vi "Static Read.vi"(8 "error in (no error)":errorcluster, 11 "Abs_Single Float in":refnum<class "Abs_Single Float.lvclass">) -> (0 "error out":errorcluster, 2 "Value":sgl, 3 "Abs_Single Float out":refnum<class "Abs_Single Float.lvclass">)   [LabVIEW 2021, in "Abs_Single Float.lvclass"]
uses:
  Abs_Single Float.lvclass
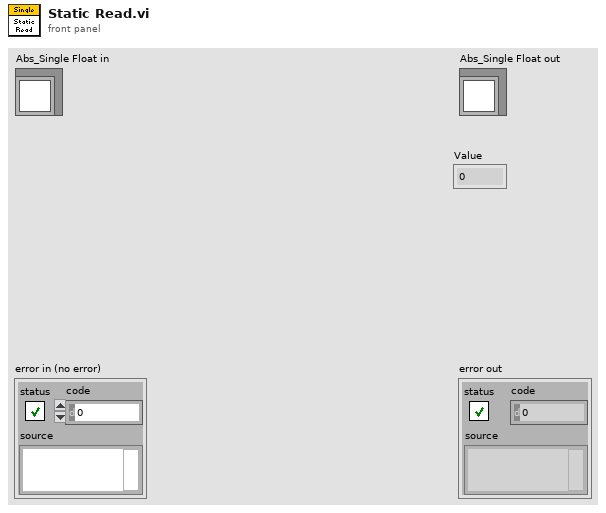
[diagram p1: front panel]
types:
  T1 = typedef "Abs_Single Float.lvclass/Type.ctl" = sgl
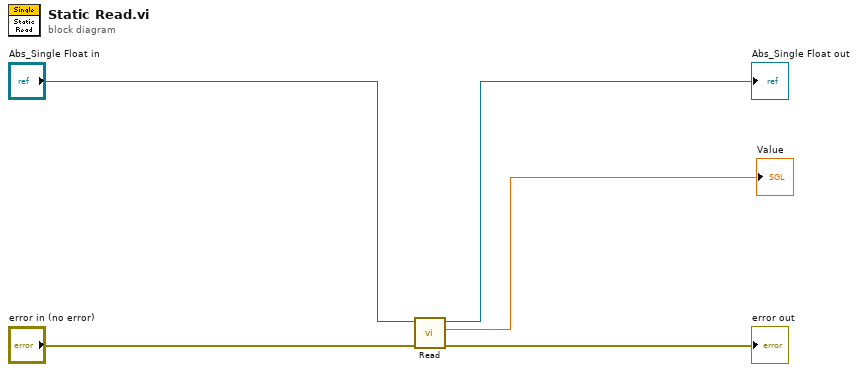
[diagram p0: block diagram]
diagram:
  n1 = call-dynamic "Read.vi"("error in (no error)"="error in (no error)", "Double Float.lvclass_340760 in"="Abs_Single Float in") -> ("error out"=→"error out":errorcluster, "Value"=→"Value":T1, "Double Float.lvclass_340760 out"=→"Abs_Single Float out":refnum<class "Abs_Single Float.lvclass">)  [unwired: 7 in]
